vi "Image Height.vi"() -> ()   [LabVIEW 2012]
panel:
  in  "Image Height":dbl
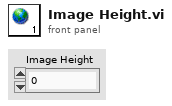
[diagram p1: front panel]
diagram:
